vi "getPolarity.vi"(0 "MultiAxisController in":refnum<class "_MultiAxisController.lvclass">, 2 "axis (in)":T1, 5 "error in (no error)":errorcluster) -> (14 "MultiAxisController out":refnum<class "_MultiAxisController.lvclass">, 16 "polarity_items (out)":T2[](array[typedef]), 19 "error out":errorcluster)   [LabVIEW 2013, in "classes.lvlib" / "_MultiAxisController.lvclass"]
doc: "Produced By:\n\n<B>Kod Integrations, LLC</B>\n4835 Marianne Drive\nMount Airy, MD 21771\nhttp://www.kodintegrations.com\nemail: info@kodintegrations.com\nphone: (240) 687-1288"
uses:
  _MultiAxisController.lvclass
  common/controls/polarity_item.ctl
  common/controls/polarity.ctl
  common/controls/axis.ctl
  common/controls/simple_actions.ctl
  Controller/_Controller.lvclass
  libraries/common.lvlib
panel:
  out "response (out)":string
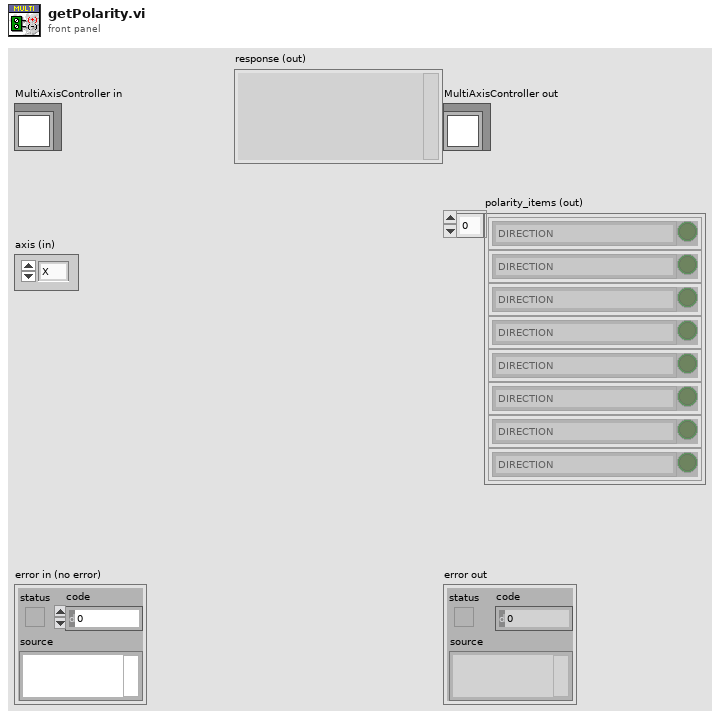
[diagram p1: front panel]
types:
  T1 = typedef "common.lvlib/axis.ctl" = enum16{"X", "Y", "Z", "U"}
  T2 = typedef "common.lvlib/polarity_item.ctl" = cluster{"item":T3, "status":bool}
  T3 = typedef "common.lvlib/polarity.ctl" = enum16{"DIRECTION", "LIMIT", "HOME", "DIG_OUT", "DIG_IN", "ENABLE_OUT", "JUMP_ERR", "LATCH", "Z-CHAN_INDEX", "ENCODER_DECODING:1X", "ENCODER_DECODING:2X", "ENCODER_DECODING:4X", "ALARM", "STANDALONE_ERR", "-", "<reserved/nc>"}
  T4 = typedef "common.lvlib/simple_actions.ctl" = enum16{"from_value", "to_value"}
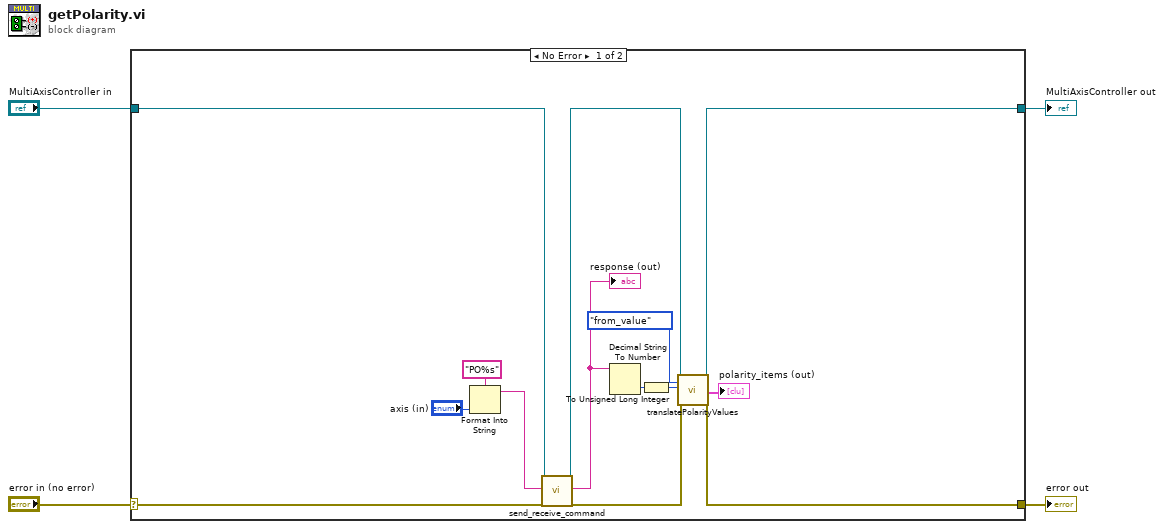
[diagram p0: block diagram]
diagram:
  n1 = case shown="No Error" "error in (no error)" {
    selector: "error in (no error)" -> [w10 w20]
    tunnel: [w8 w20] -> w3
    tunnel: [w5 w19] -> w1
    tunnel: "MultiAxisController in" -> [w7 w19]
    frame No Error {
      n2 = Format Into String(format string="PO%s" ("ASCII Command (in)"), "axis (in)") -> (resulting string=w11:string)  [unwired: 2 in, 1 out]
      n3 = call "send_receive_command.vi"("reference (in)"=w7, "ASCII Command (in)"=w11, "error in (no error)"=w10) -> ("reference (out)"=w6:refnum<class "_MultiAxisController.lvclass">, "response (out)"=w18:string, "error out"=w9:errorcluster)  [unwired: 12 in, 2 out]
      "response (out)" <- w18
      n4 = Decimal String To Number(string=w18) -> (number=w16:i32)  [unwired: 2 in, 1 out]
      n5 = To Unsigned Long Integer(number=w16) -> (unsigned 32bit integer=w14:u32)
      n6 = call-dynamic "translatePolarityValues.vi"("Controller in"=w6, "simple_actions"=simple_actions."from_value", "polarity_value (in)"=w14, "error in (no error)"=w9) -> ("Controller out"=w5:refnum<class "_MultiAxisController.lvclass">, "polarity_items (out)"=→"polarity_items (out)":T2[], "error out"=w8:errorcluster)  [unwired: 12 in, 1 out]
    }
    frame Error {
    }
  }
  "error out" <- w3
  "MultiAxisController out" <- w1
